vi "Read ERD Example.vi"(0 "GEA Inputs":T1 {"Destination" format="%.0x"; "Source" format="%.0x"}, 1 "Read Timeout (ms)":u32=500, 2 "Device Selected":i32, 5 "Retry Count":i32=5, 6 "Read ERD List":T2[](array[typedef]) {"ERD Number" format="%.0x"}, 11 "Error In":errorcluster, 13 "Verify ERD Response?":bool) -> (4 "Data Returned":string, 7 "ERD Data Out":T3[](array[typedef]) {"ERD Number" format="%.0x"}, 15 "Error Out":errorcluster)   [LabVIEW 2014]
doc: "This standalone VI reads the next message on the GEA2 bus OR waits until it receives a message with the command or data you specify. (.* = anything)"
uses:
  type defs/ERD Read Data Out.ctl
  type defs/ERD Read Data In.ctl
  type defs/Source_Destination.ctl
  library/GEA2_Toolkit.lvlib
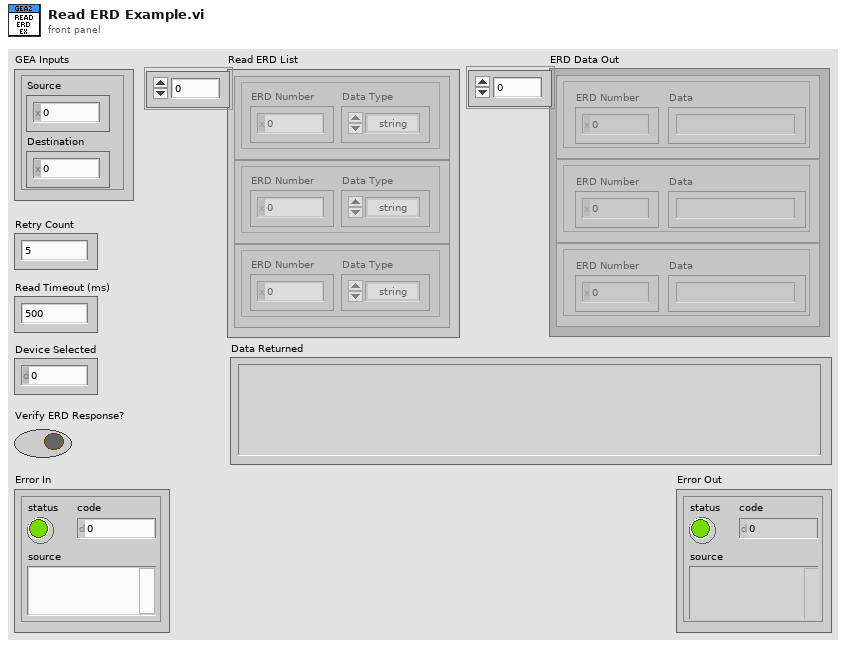
[diagram p1: front panel]
types:
  T1 = typedef "GEA2_Toolkit.lvlib/Source_Destination.ctl" = cluster{"Source":u8, "Destination":u8}
  T2 = typedef "GEA2_Toolkit.lvlib/ERD Read Data In.ctl" = cluster{"ERD Number":u16, "Data Type":enum16{"string", "boolean", "uint8_t", "uint16_t", "uint32_t", "uint64_t"}}
  T3 = typedef "GEA2_Toolkit.lvlib/ERD Read Data Out.ctl" = cluster{"ERD Number":u16, "Data":string}
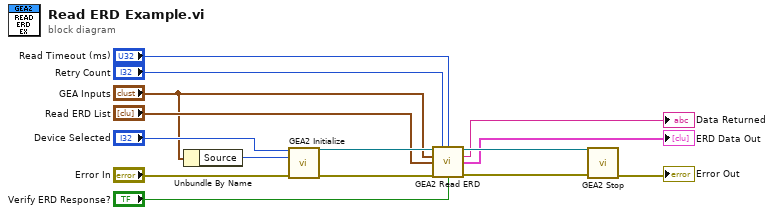
[diagram p0: block diagram]
diagram:
  n1 = Unbundle By Name("GEA Inputs") -> ("Source"=w1:u8)
  n2 = call "GEA2 Initialize.vi"("Board Index"="Device Selected", "Source Address"=w1, "error in"="Error In") -> ("GEA2 Reference Out"=w5:refnum<k24>, "error out"=w13:errorcluster)  [unwired: 10 in, 1 out]
  n3 = call "GEA2 Read ERD.vi"("GEA2 Reference In"=w5, "Retry Count"="Retry Count", "Read Timeout (ms)"="Read Timeout (ms)", "GEA Inputs"="GEA Inputs", "Read ERD List"="Read ERD List", "Error In"=w13, "Verify ERD Response?"="Verify ERD Response?") -> ("GEA2 Reference Out"=w14:refnum<k24>, "Raw Data Out"=→"Data Returned":string, "ERD Data Out"=→"ERD Data Out":T3[], "Error Out"=w15:errorcluster)  [unwired: 5 in]
  n4 = call "GEA2 Stop.vi"("GEA2 Reference In"=w14, "Error In"=w15) -> ("Error Out"=→"Error Out":errorcluster)  [unwired: 13 in]
